vi "Mouse Gesture Handler with Messenger Channel.vi"() -> ()   [LabVIEW 2019]
doc: "This VI illustrates the use of a Messenger channel to communicate UI gestures from a mouse tracking loop to a slower picture rendering loop to implement a simple picture-control-based editor."
uses:
  <vilib>/Utility/miscctls.llb/LVRectTypeDef.ctl
  <extravilib>/ChannelInstances/Messenger2-class'Gesture Wrapper'/Write With Abort.vi
  <extravilib>/ChannelInstances/Messenger2-class'Gesture Wrapper'/Read With Abort.vi
  Gesture Wrapper/Gesture Wrapper.lvclass
  e:/builds/penguin/labview/branches/2019/dev/dist/vi.lib/ChannelSupport/Channel Message/Channel Message.lvclass
  <extravilib>/ChannelInstances/Messenger2-class'Gesture Wrapper'/Instantiate.vi
  <extravilib>/ChannelInstances/Messenger2-class'Gesture Wrapper'/Endpoint.vi
  Gesture/Gesture.lvclass
  Blob/Blob.lvclass
  <extravilib>/ChannelInstances/Messenger2-class'Gesture Wrapper'.lvlib
panel:
  in  "Stop":bool
  out "canvas":picture
  # "Overview: \nDemonstrates the use of the Messenger channel to communicate gestures from a mouse tracking loop to a picture rendering loop in order to implement a simple picture control based editor.\n\nThis example assumes you are already familiar with channels. If you are not, you may want to review this example first:\nexamples\\Channels\\Basics\\Channel Basics.lvproj\n\nInstructions:\n1. Run the VI.\n2. Click the square and drag it around within the canvas.\n3. Click Stop to stop the VI.\n4. See the block diagram for more information about the use of the Messenger channel."
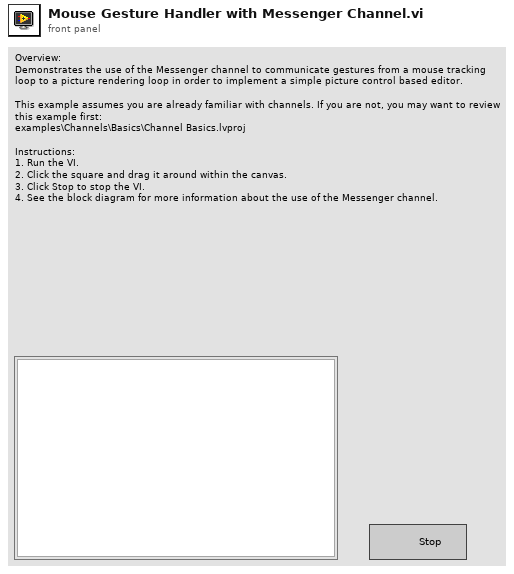
[diagram p1: front panel]
types:
  T1 = typedef "LVRectTypeDef.ctl" = cluster{"Left":i16, "Top":i16, "Right":i16, "Bottom":i16}
  T2 = typedef "LVMouseTypeDef.ctl" = cluster{"Mouse Position":cluster{"X":i32, "Y":i32}, "Mouse Modifiers":cluster{"Button Down":bool, "Shift Mod":bool, "Menu Mod":bool, "Option Mod":bool}}
  T3 = typedef "Messenger2-class'Gesture Wrapper'.lvlib/))Channel.ctl" = refnum<queue>
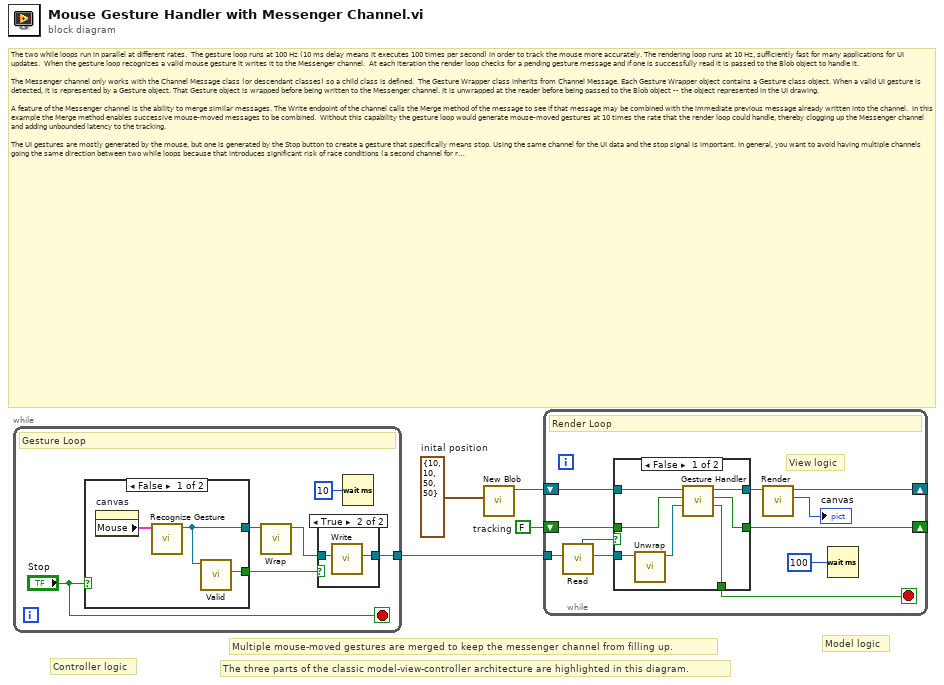
[diagram p0: block diagram]
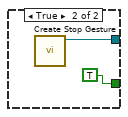
[diagram p3: hidden frame]
diagram:
  w1 = T1 {"Left"=10, "Top"=10, "Right"=50, "Bottom"=50}  # inital position
  w4 = FALSE  # tracking
  # "The three parts of the classic model-view-controller architecture are highlighted in this diagram."
  # "Model logic"
  # "Controller logic"
  # "The two while loops run in parallel at different rates.  The gesture loop runs at 100 Hz (10 ms delay means it executes 100 times per second) in order to track the mouse more accurately. The rendering loop runs at 10 Hz, sufficiently fast for many applications for UI updates.  When the gesture loop recognizes a valid mouse gesture it writes it to the Messenger channel.  At each iteration the render loop checks for a pending gesture message and if one is successfully read it is passed to the Blob object to handle it.\n\nThe Messenger channel only works with the Channel Message class (or descendant classes) so a child class is defined.  The Gesture Wrapper class inherits from Channel Message. Each Gesture Wrapper object contains a Gesture class object. When a valid UI gesture is detected, it is represented by a Gesture object. That Gesture object is wrapped before being written to the Messenger channel. It is unwrapped at the reader before being passed to the Blob object -- the object represented in the UI drawing.\n\nA feature of the Messenger channel is the ability to merge similar messages. The Write endpoint of the channel calls the Merge method of the message to see if that message may be combined with the immediate previous message already written into the channel.  In this example the Merge method enables successive mouse-moved messages to be combined.  Without this capability the gesture loop would generate mouse-moved gestures at 10 times the rate that the render loop could handle, thereby clogging up the Messenger channel and adding unbounded latency to the tracking.\n\nThe UI gestures are mostly generated by the mouse, but one is generated by the Stop button to create a gesture that specifically means stop. Using the same channel for the UI data and the stop signal is important. In general, you want to avoid having multiple channels going the same direction between two while loops because that introduces significant risk of race conditions (a second channel for reverse direction communication is fine). Another shipping example demonstrates the issue:\nexamples\\Channels\\Parallel Channels Problem\\Parallel Channels Problem.lvproj"
  # "Multiple mouse-moved gestures are merged to keep the messenger channel from filling up."
  n1 = while {
    tunnel: [w6] -> w2
    stop <- "Stop" stop-if-true
    # "Gesture Loop"
    n2 = case shown="False" "Stop" {
      tunnel: [w15 TRUE ("valid")] -> w5
      tunnel: [w13 w17] -> w9
      frame False {
        n3 = property on="canvas" class="Pict"() -> ("Mouse"=w14:T2)  [unwired: 2 in, 2 out]
        n4 = call "Recognize Gesture.vi"("mouse"=w14) -> ("gesture"=w13:refnum<class "Gesture.lvclass">)  [unwired: 10 in]
        n5 = call-dynamic "Valid.vi"("gesture in"=w13) -> ("valid"=w15:bool)  [unwired: 10 in]
      }
      frame True {
        n6 = call "Create Stop Gesture.vi"() -> ("Gesture out"=w17:refnum<class "Gesture.lvclass">)  [unwired: 11 in]
      }
    }
    n7 = call "Wrap.vi"("gesture"=w9) -> ("Gesture Wrapper"=w10:refnum<class "Gesture Wrapper.lvclass">)  [unwired: 10 in]
    n8 = case shown="True" w5 {
      tunnel: w10 -> [_ w12]
      tunnel: [_ w11] -> w6
      frame False {
      }
      frame True {
        n9 = call <extravilib>:"Write.vi"("element"=w12) -> ("channel"=w11:T3)  [unwired: 8 in, 2 out]
      }
    }
    n10 = Wait (ms)(milliseconds to wait=u32 10) -> ()  [unwired: 1 out]
  }
  n11 = call "New Blob.vi"("rect"=w1) -> ("Blob out"=w3:refnum<class "Blob.lvclass">)  [unwired: 10 in]
  n12 = while {
    shift-right: [w28] -> _
    shift-left: w3 -> [w27]
    shift-right: [w24] -> _
    shift-left: w4 -> [w25]
    tunnel: w2 -> [w20]
    stop <- w18 stop-if-true
    # "View logic"
    # "Render Loop"
    n13 = call <extravilib>:"Read.vi"("channel"=w20) -> ("element"=w21:refnum<class "Gesture Wrapper.lvclass">, "timed out?"=w22:bool)  [unwired: 8 in, 1 out]
    n14 = case shown="False" w22 {
      tunnel: w21 -> [w33 _]
      tunnel: w27 -> [w35 w37]
      tunnel: [w34 w37] -> w26
      tunnel: w25 -> [w32 w36]
      tunnel: [w30 w36] -> w24
      tunnel: [w29 _] -> w18
      frame False {
        n15 = call "Unwrap.vi"("Channel Message"=w33) -> ("gesture"=w31:refnum<class "Gesture.lvclass">)  [unwired: 10 in]
        n16 = call-dynamic "Gesture Handler.vi"("gesture"=w31, "tracking in"=w32, "Blob in"=w35) -> ("stop?"=w29:bool, "tracking out"=w30:bool, "Blob out"=w34:refnum<class "Blob.lvclass">)  [unwired: 6 in]
      }
      frame True {
      }
    }
    n17 = call-dynamic "Render.vi"("Blob in"=w26) -> ("image"=→"canvas":picture, "Blob out"=w28:refnum<class "Blob.lvclass">)  [unwired: 9 in]
    n18 = Wait (ms)(milliseconds to wait=u32 100) -> ()  [unwired: 1 out]
  }
